vi "PIDOutput2MotorOutput.vi"(11 "PID Output":dbl) -> (1 "Dir2":bool, 2 "Dir1":bool, 3 "Duty Cycle":dbl)   [LabVIEW 2021]
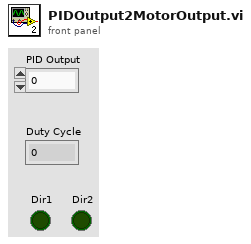
[diagram p1: front panel]
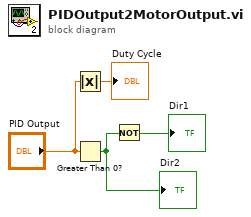
[diagram p0: block diagram]
diagram:
  n1 = Absolute Value(x="PID Output") -> (abs(x)=→"Duty Cycle":dbl)
  n2 = Greater Than 0?(x="PID Output") -> (x > 0?=w1:bool)
  "Dir2" <- w1
  n3 = Not(x=w1) -> (.not. x?=→"Dir1":bool)
